vi "Read Default Funnel Cluster.vi"(8 "error in (no error)":errorcluster, 11 "Funnel Settings in":refnum<class "Funnel Settings.lvclass">) -> (0 "error out":errorcluster, 2 "Default Funnel":T1, 3 "Funnel Settings out":refnum<class "Funnel Settings.lvclass">)   [LabVIEW 2019, in "Funnel Settings.lvclass"]
uses:
  Funnel Settings.lvclass
  Typedefs/Default Funnel Cluster.ctl
  Funnel Settings.lvclass/Funnel Settings.ctl
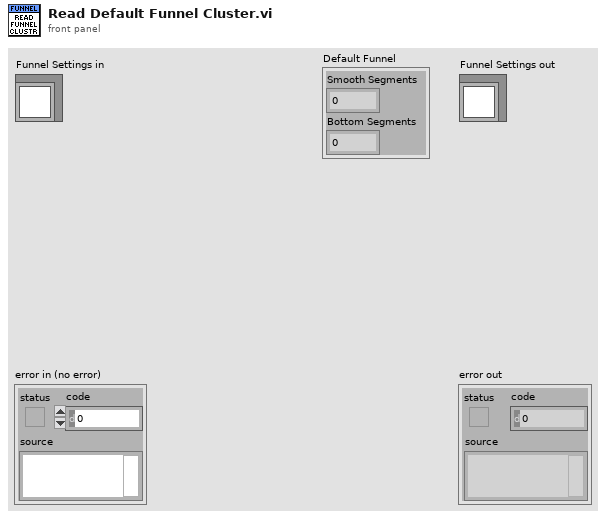
[diagram p1: front panel]
types:
  T1 = typedef "Funnel Settings.lvclass/Default Funnel Cluster.ctl" = cluster{"Smooth Segments":dbl, "Bottom Segments":dbl}
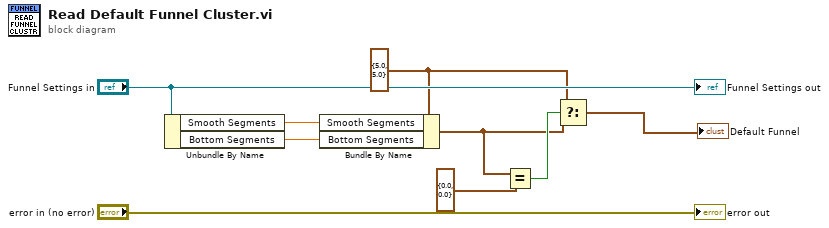
[diagram p0: block diagram]
diagram:
  w3 = T1 {"Smooth Segments"=5.0, "Bottom Segments"=5.0} ("cluster")
  n1 = Unbundle By Name("Funnel Settings in") -> ("Smooth Segments"=w7:dbl, "Bottom Segments"=w6:dbl)
  n2 = Bundle By Name(cluster=w3, "Smooth Segments"=w7, "Bottom Segments"=w6) -> (w2:T1)
  n3 = Equal?(x=w2, y=T1 {"Smooth Segments"=0.0, "Bottom Segments"=0.0} ("output cluster")) -> (x = y?=w4:bool)
  n4 = Select(t=w3, s=w4, f=w2) -> (s? t:f=→"Default Funnel":T1)
  "error out" <- "error in (no error)"
  "Funnel Settings out" <- "Funnel Settings in"
